vi "zadSpr_002_PH.vi"() -> ()   [LabVIEW 2021]
panel:
  out "Button 2":bool
  out "Boolean 3":bool=TRUE
  out "String":string="pierwszy cluster"
  out "Button":bool=TRUE
  out "Array":i16[](array[numeric])=[2020, 2020, 2020, 2020, 2020]
  out "Boolean 2":bool=TRUE
  out "Array 2":i16[](array[numeric])=[2020, 2020, 2020, 2020, 2020]
  in  "Cluster":T1={"Array"=[2020, 2020, 2020, 2020, 2020], "Button"=TRUE, "String"="pierwszy cluster", "Button 2"=FALSE}
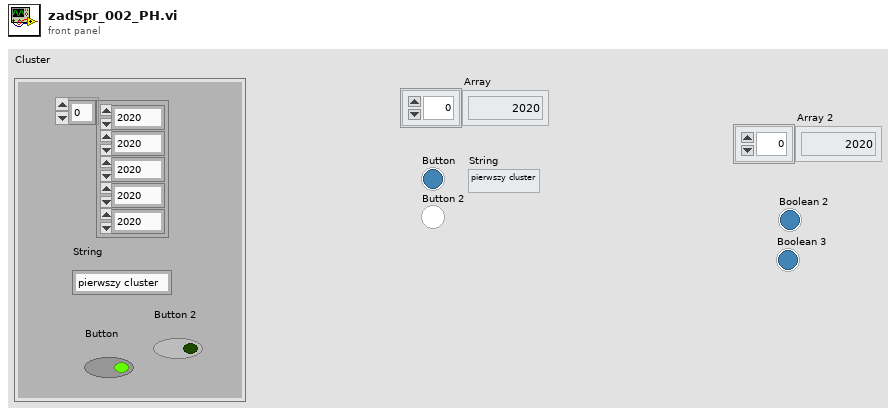
[diagram p1: front panel]
types:
  T1 = cluster{"Array":i16[], "Button":bool, "String":string, "Button 2":bool}
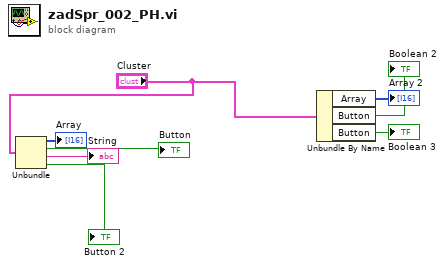
[diagram p0: block diagram]
diagram:
  n1 = Unbundle("Cluster") -> ("Array"=→"Array":i16[], "Button"=→"Button":bool, "String"=→"String":string, "Button 2"=→"Button 2":bool)
  n2 = Unbundle By Name("Cluster") -> ("Array"=→"Array 2":i16[], "Button"=→"Boolean 2":bool, "Button"=→"Boolean 3":bool)
